vi "instrument_cluster.vi"() -> ()   [LabVIEW 2014]
uses:
  stateCtl.ctl
  <vilib>/Instr/_visa.llb/VISA Configure Serial Port (Instr).vi
  <vilib>/Utility/miscctls.llb/LVTextColorsTypeDef.ctl
  <vilib>/Utility/miscctls.llb/LVSelectionTypeDef.ctl
  <vilib>/Utility/miscctls.llb/LVFontTypeDef.ctl
  <vilib>/Utility/miscctls.llb/LVForegroundBackgroundColorsTypeDef.ctl
panel:
  out "S5":string
  out "S4":string
  out "S3":string
  out "S2":string
  out "S1":string
  out "S0":string
  in  "Text.Font 4":T1={"Font Name"="Arial", "Size"=0, "Bold"=FALSE, "Italic"=FALSE, "Underline"=FALSE, "Strikeout"=FALSE, "Color"=16776746}
  in  "Text.Text Colors 2":T2={"Text Color"=0, "Background Color"=3153414}
  in  "Text.Selection 2":T3
  in  "Text.Font 2":T1={"Font Name"="Arial", "Size"=55, "Bold"=FALSE, "Italic"=FALSE, "Underline"=FALSE, "Strikeout"=FALSE, "Color"=16776746}
  in  "Text.Colors 2":T4={"Foreground Color"=0, "Background Color"=3153414}
  in  "Text.Text Colors 3":T2={"Text Color"=0, "Background Color"=3153414}
  in  "Text.Selection 3":T3
  in  "Text.Font 3":T1={"Font Name"="Arial", "Size"=0, "Bold"=FALSE, "Italic"=FALSE, "Underline"=FALSE, "Strikeout"=FALSE, "Color"=16776746}
  in  "Text.Colors 3":T4={"Foreground Color"=0, "Background Color"=3153414}
  in  "Text.Colors":T4={"Foreground Color"=0, "Background Color"=3153414}
  in  "Text.Font":T1={"Font Name"="Arial", "Size"=15, "Bold"=FALSE, "Italic"=FALSE, "Underline"=FALSE, "Strikeout"=FALSE, "Color"=16776746}
  in  "Text.Selection":T3
  in  "Text.Text Colors":T2={"Text Color"=0, "Background Color"=3153414}
  out "exitLed":bool
  out "statusBar":string="     "
  in  "startButton":bool
  out "stopLed":bool
  out "startLed":bool
  in  "VISA Serial Port":refnum<visa-resource-name>
  in  "exitButton":bool
  in  "stopButton":bool
  # "String G"
  # "Gear String"
  # "Travelled Distance String"
  # "Pedal Position String"
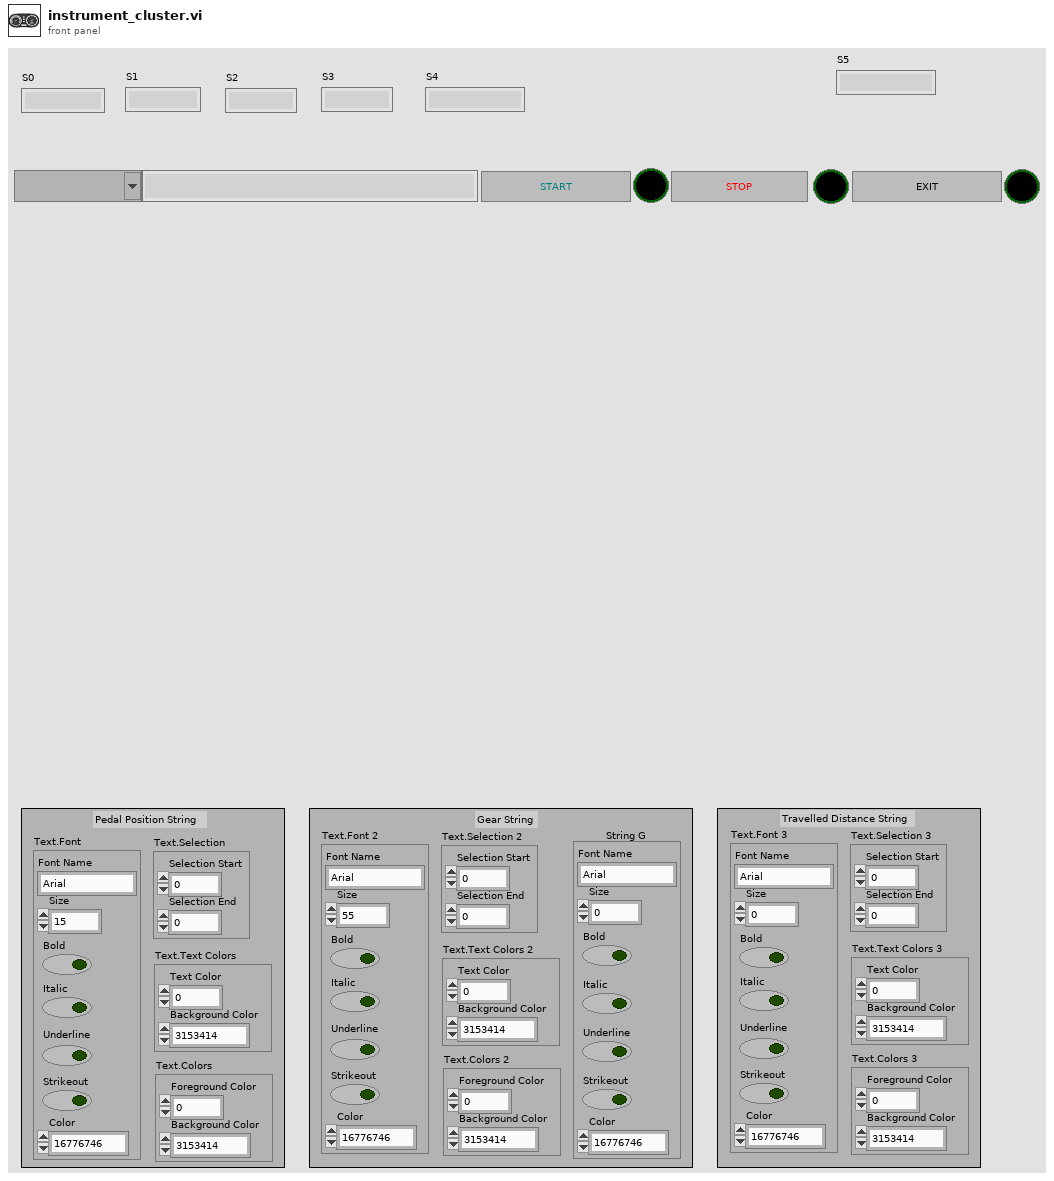
[diagram p1: front panel]
types:
  T1 = typedef "LVFontTypeDef.ctl" = cluster{"Font Name":string, "Size":u16, "Bold":bool, "Italic":bool, "Underline":bool, "Strikeout":bool, "Color":u32}
  T2 = typedef "LVTextColorsTypeDef.ctl" = cluster{"Text Color":u32, "Background Color":u32}
  T3 = typedef "LVSelectionTypeDef.ctl" = cluster{"Selection Start":u32, "Selection End":u32}
  T4 = typedef "LVForegroundBackgroundColorsTypeDef.ctl" = cluster{"Foreground Color":u32, "Background Color":u32}
  T5 = typedef "stateCtl.ctl" = enum16{"init", "ready", "running", "stopped", "exit"}
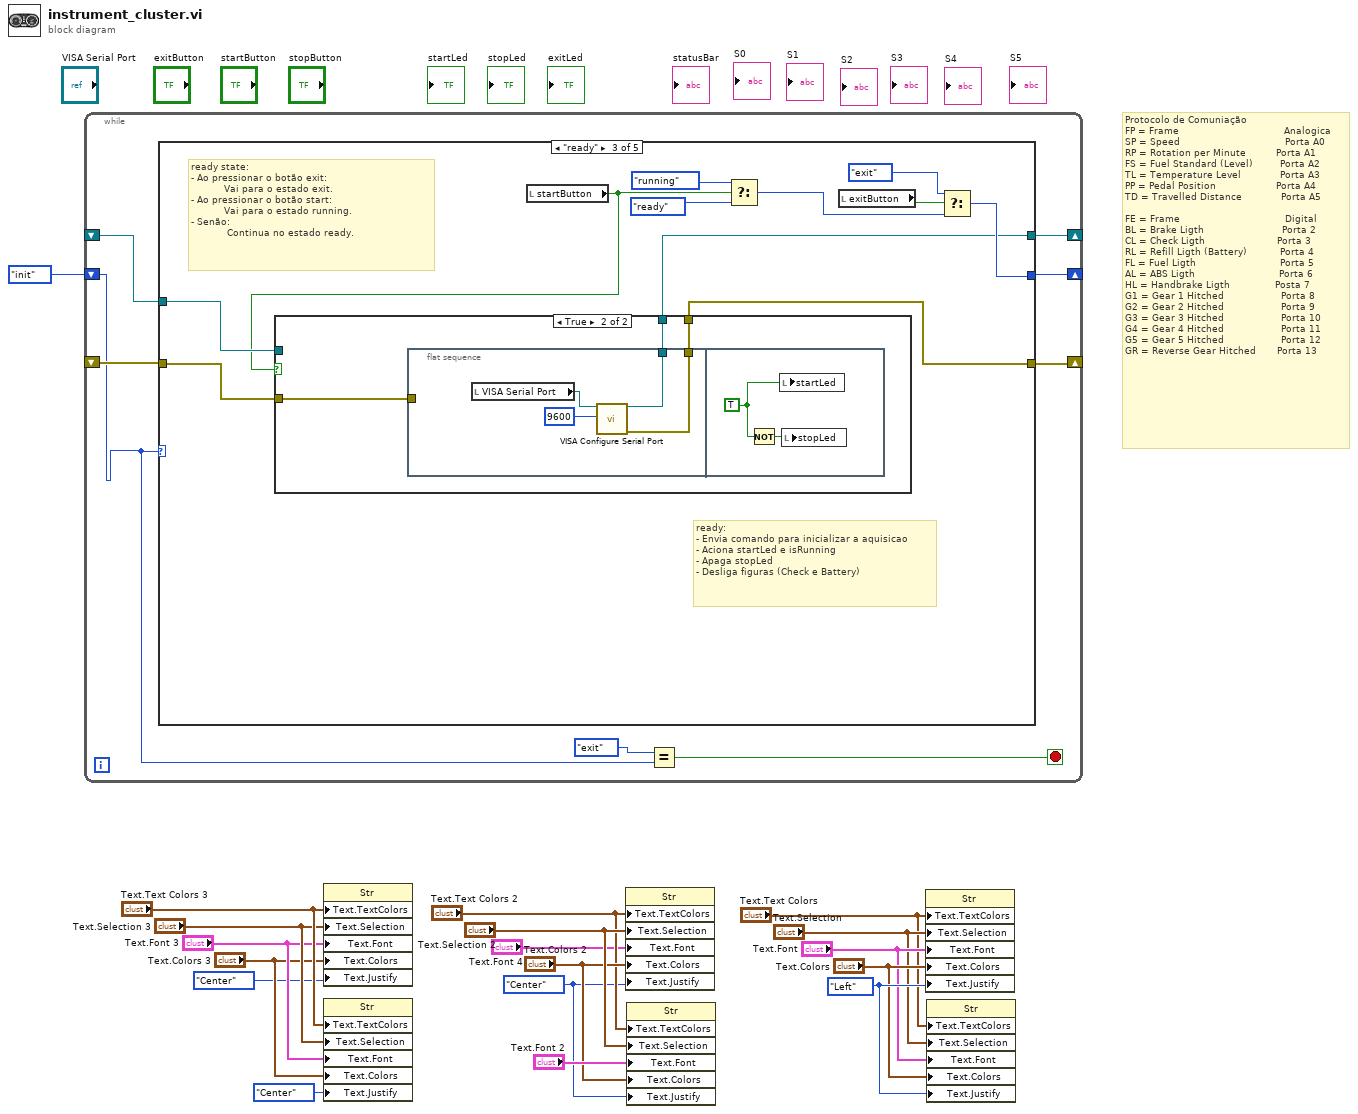
[diagram p0: block diagram]
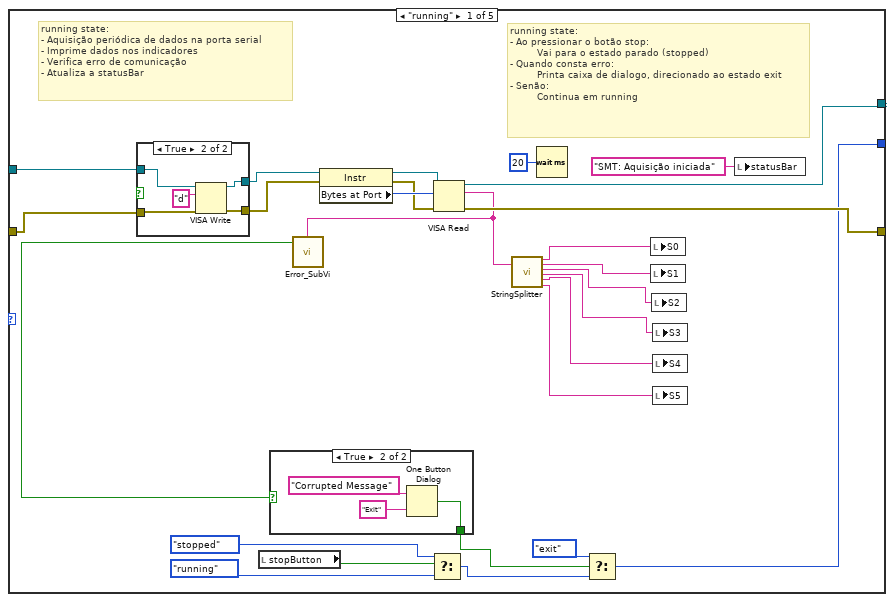
[diagram p2: hidden frame]
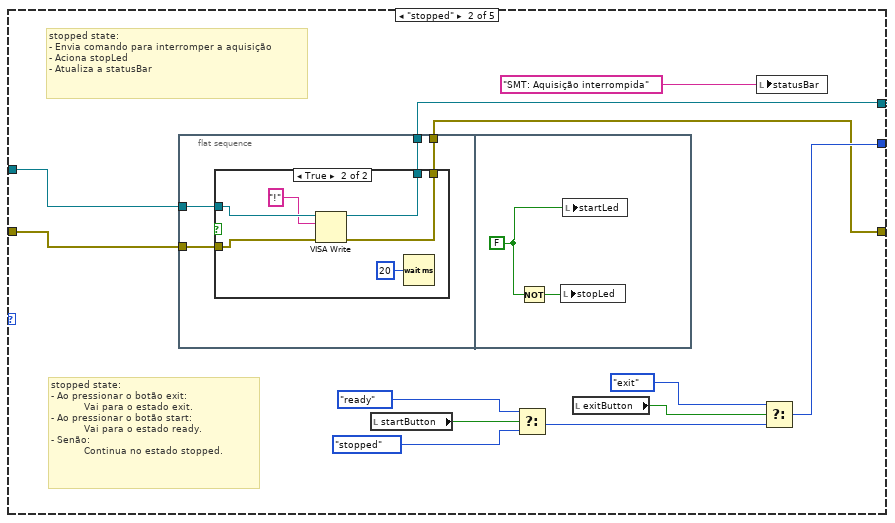
[diagram p5: hidden frame]
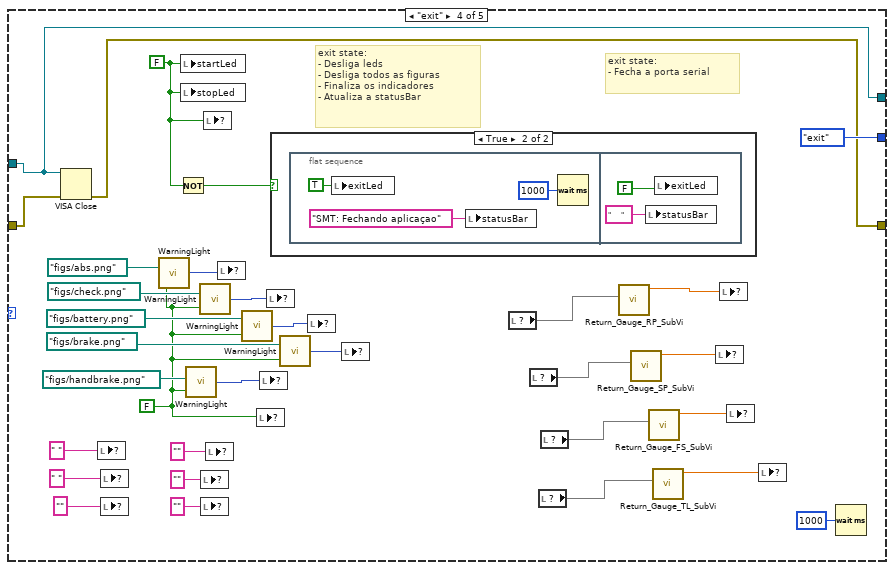
[diagram p8: hidden frame]
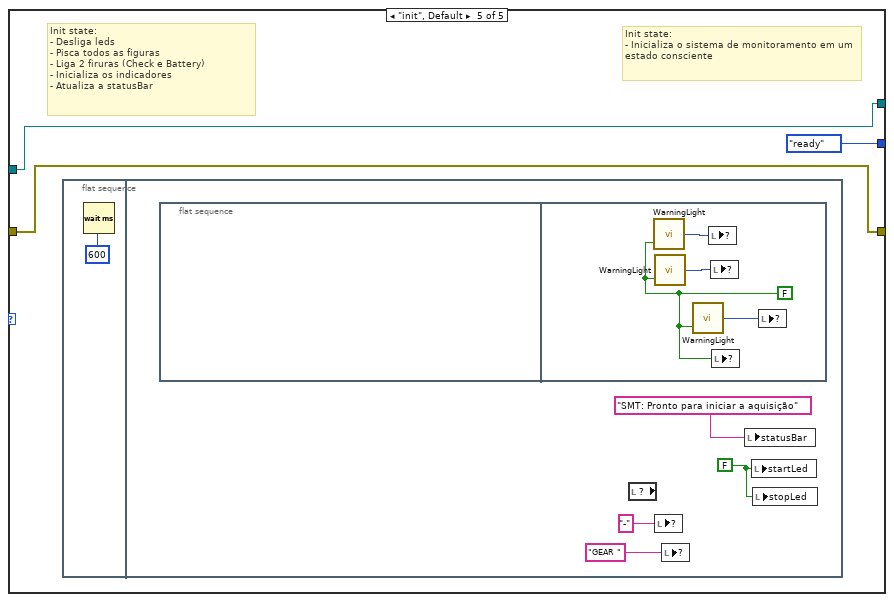
[diagram p10: hidden frame]
diagram:
  w1 = enum16{"Left", "Center", "Right"}."Center" ("Text.Justification")
  w23 = enum16{"Left", "Center", "Right"}."Left" ("Text.Justification")
  # "Protocolo de Comuniação \nFP = Frame                                   Analogica  \nSP = Speed                                   Porta A0\nRP = Rotation per Minute          Porta A1\nFS = Fuel Standard (Level)         Porta A2\nTL = Temperature Level             Porta A3\nPP = Pedal Position                    Porta A4\nTD = Travelled Distance             Porta A5\n\nFE = Frame                                   Digital \nBL = Brake Ligth                          Porta 2 \nCL = Check Ligth                        Porta 3\nRL = Refill Ligth (Battery)           Porta 4\nFL = Fuel Ligth                            Porta 5 \nAL = ABS Ligth                            Porta 6\nHL = Handbrake Ligth               Posta 7\nG1 = Gear 1 Hitched                   Porta 8\nG2 = Gear 2 Hitched                   Porta 9\nG3 = Gear 3 Hitched                   Porta 10\nG4 = Gear 4 Hitched                   Porta 11\nG5 = Gear 5 Hitched                   Porta 12\nGR = Reverse Gear Hitched       Porta 13"
  n1 = while {
    shift-right: [w27] -> _
    shift-left: _ -> [w31]
    shift-right: [w32] -> _
    shift-left: _ -> [w30]
    shift-right: [w28] -> _
    shift-left: stateCtl."init" ("state") -> [w25]
    stop <- w26 stop-if-true
    n2 = case shown="\"ready\"" w25 {
      tunnel: [w51 w74 w98 w150 w160] -> w27
      tunnel: [w50 w75 w97 w151 w159] -> w32
      tunnel: [w43 w79 w101 stateCtl."exit" ("state") stateCtl."ready" ("state")] -> w28
      tunnel: w31 -> [w45 w77 w99 w150 w160]
      tunnel: w30 -> [w46 w76 w100 w152 w159]
      frame "running" {
        # "running state:\n- Ao pressionar o botão stop: \n         Vai para o estado parado (stopped)\n- Quando consta erro:\n         Printa caixa de dialogo, direcionado ao estado exit  \n- Senão:          \n         Continua em running"
        # "running state:\n- Aquisição periódica de dados na porta serial\n- Imprime dados nos indicadores\n- Verifica erro de comunicação\n- Atualiza a statusBar"
        n3 = case shown="True" {
          selector: _ -> [_ _]
          tunnel: [w64 w68] -> w48
          tunnel: [w63 w67] -> w47
          tunnel: w46 -> [w64 w66]
          tunnel: w45 -> [w63 w65]
          frame False {
          }
          frame True {
            n4 = VISA Write(VISA resource name=w65, write buffer="d", error in (no error)=w66) -> (VISA resource name out=w67:refnum<visa-resource-name>, error out=w68:errorcluster)  [unwired: 1 out]
          }
        }
        n5 = local read "stopButton"() -> (w56:bool)
        n6 = property class="Instr"(reference=w47, error in=w48) -> (reference out=w52:refnum<visa-resource-name>, error out=w53:errorcluster, "Bytes at Port"=w54:u32)
        n7 = Select(t=stateCtl."stopped" ("state"), s=w56, f=stateCtl."running" ("state")) -> (s? t:f=w42:T5)
        n8 = VISA Read(VISA resource name=w52, byte count=w54, error in (no error)=w53) -> (VISA resource name out=w51:refnum<visa-resource-name>, read buffer=w39:string, error out=w50:errorcluster)  [unwired: 1 out]
        n9 = call "Error_SubVi.vi"("string"=w39) -> ("error"=w40:bool)  [unwired: 10 in]
        n10 = case shown="True" w40 {
          selector: w40 -> [w59 _]
          tunnel: [w59 w60] -> w41
          frame False {
          }
          frame True {
            n11 = One Button Dialog(message="Corrupted Message", button name ("OK")="Exit") -> (true=w60:bool)
          }
        }
        n12 = call "StringSplitter.vi"("Input String"=w39) -> ("S0"=w38:string, "S1"=w37:string, "S2"=w36:string, "S3"=w35:string, "S4"=w34:string, "S5"=w33:string)  [unwired: 13 in]
        n13 = Wait (ms)(milliseconds to wait=u32 20) -> ()  [unwired: 1 out]
        n14 = Select(t=stateCtl."exit" ("state"), s=w41, f=w42) -> (s? t:f=w43:T5)
        n15 = local write "S0"(w38) -> ()
        n16 = local write "S1"(w37) -> ()
        n17 = local write "S2"(w36) -> ()
        n18 = local write "S3"(w35) -> ()
        n19 = local write "S4"(w34) -> ()
        n20 = local write "S5"(w33) -> ()
        n21 = local write "statusBar"("SMT: Aquisição iniciada" ("statusBar")) -> ()
      }
      frame "stopped" {
        # "stopped state:\n- Ao pressionar o botão exit: \n           Vai para o estado exit.\n- Ao pressionar o botão start:\n           Vai para o estado ready.\n- Senão:\n           Continua no estado stopped."
        # "stopped state:\n- Envia comando para interromper a aquisição\n- Aciona stopLed\n- Atualiza a statusBar"
        n22 = flat-sequence {
          tunnel: w77 -> [w85]
          tunnel: w76 -> [w84]
          tunnel: [w83] -> w75
          tunnel: [w82] -> w74
          frame #0 {
            n23 = case shown="True" {
              selector: _ -> [_ _]
              tunnel: w85 -> [w87 w93]
              tunnel: w84 -> [w86 w92]
              tunnel: [w86 w88] -> w83
              tunnel: [w87 w90] -> w82
              frame False {
              }
              frame True {
                n24 = VISA Write(VISA resource name=w93, write buffer="!", error in (no error)=w92) -> (VISA resource name out=w90:refnum<visa-resource-name>, error out=w88:errorcluster)  [unwired: 1 out]
                n25 = Wait (ms)(milliseconds to wait=u32 20) -> ()  [unwired: 1 out]
              }
            }
          }
          frame #1 {
            w95 = FALSE ("Boolean")
            n26 = Not(x=w95) -> (.not. x?=w94:bool)
            n27 = local write "stopLed"(w94) -> ()
            n28 = local write "startLed"(w95) -> ()
          }
        }
        n29 = local read "startButton"() -> (w73:bool)
        n30 = Select(t=stateCtl."ready" ("state"), s=w73, f=stateCtl."stopped" ("state")) -> (s? t:f=w80:T5)
        n31 = local read "exitButton"() -> (w72:bool)
        n32 = local write "statusBar"("SMT: Aquisição interrompida" ("statusBar")) -> ()
        n33 = Select(t=stateCtl."exit" ("state"), s=w72, f=w80) -> (s? t:f=w79:T5)
      }
      frame "ready" {
        # "ready state:\n- Ao pressionar o botão exit: \n           Vai para o estado exit.\n- Ao pressionar o botão start:\n           Vai para o estado running.\n- Senão:\n            Continua no estado ready."
        # "ready:\n- Envia comando para inicializar a aquisicao\n- Aciona startLed e isRunning\n- Apaga stopLed\n- Desliga figuras (Check e Battery)"
        n34 = local read "startButton"() -> (w96:bool)
        n35 = case shown="True" w96 {
          tunnel: [w108 w109] -> w98
          tunnel: [w107 w110] -> w97
          tunnel: w99 -> [w108 _]
          tunnel: w100 -> [w107 w111]
          frame False {
          }
          frame True {
            n36 = flat-sequence {
              tunnel: w111 -> [_]
              tunnel: [w113] -> w110
              tunnel: [w112] -> w109
              frame #0 {
                n37 = local read "VISA Serial Port"() -> (w114:refnum<visa-resource-name>)
                n38 = call-poly "VISA Configure Serial Port"("VISA resource name"=w114, "baud rate (9600)"=u32 9600) -> ("VISA resource name out"=w112:refnum<visa-resource-name>, "error out"=w113:errorcluster)  [unwired: 12 in]
              }
              frame #1 {
                w117 = TRUE ("Boolean")
                n39 = Not(x=w117) -> (.not. x?=w116:bool)
                n40 = local write "startLed"(w117) -> ()
                n41 = local write "stopLed"(w116) -> ()
              }
            }
          }
        }
        n42 = Select(t=stateCtl."running" ("state"), s=w96, f=stateCtl."ready" ("state")) -> (s? t:f=w102:T5)
        n43 = local read "exitButton"() -> (w104:bool)
        n44 = Select(t=stateCtl."exit" ("state"), s=w104, f=w102) -> (s? t:f=w101:T5)
      }
      frame "exit" {
        w124 = FALSE
        w141 = FALSE ("startLed")
        # "exit state:\n- Desliga leds\n- Desliga todos as figuras\n- Finaliza os indicadores\n- Atualiza a statusBar"
        # "exit state:\n- Fecha a porta serial"
        n45 = VISA Close(VISA resource name=w150, error in (no error)=w152) -> (error out=w151:errorcluster)
        n46 = local write item#-1(" " ("String Gear")) -> ()
        n47 = local write item#-1(" " ("String TD")) -> ()
        n48 = local write item#-1("" ("String PP")) -> ()
        n49 = call "WarningLight.vi"("Boolean"=w124, "Path"=path "figs/abs.png" ("path to PNG file")) -> ("new picture"=w145:picture)
        n50 = Not(x=w141) -> (.not. x?=w142:bool)
        n51 = local write "startLed"(w141) -> ()
        n52 = local write "stopLed"(w141) -> ()
        n53 = call "WarningLight.vi"("Boolean"=w124, "Path"=path "figs/handbrake.png" ("path to PNG file")) -> ("new picture"=w132:picture)
        n54 = call "WarningLight.vi"("Boolean"=w124, "Path"=path "figs/check.png" ("path to PNG file")) -> ("new picture"=w146:picture)
        n55 = local write item#-1("" ("TD")) -> ()
        n56 = local write item#-1("" ("pedalPosition")) -> ()
        n57 = local write item#-1(w141) -> ()
        n58 = local write item#-1("" ("Gear")) -> ()
        n59 = local write item#-1(w145) -> ()
        n60 = call "WarningLight.vi"("Boolean"=w124, "Path"=path "figs/battery.png" ("path to PNG file")) -> ("new picture"=w147:picture)
        n61 = local write item#-1(w124) -> ()
        n62 = local write item#-1(w132) -> ()
        n63 = local write item#-1(w146) -> ()
        n64 = case shown="True" w142 {
          frame False {
          }
          frame True {
            n65 = flat-sequence {
              frame #0 {
                n66 = local write "exitLed"(TRUE ("exitLed")) -> ()
                n67 = local write "statusBar"("SMT: Fechando aplicaçao" ("statusBar")) -> ()
                n68 = Wait (ms)(milliseconds to wait=u32 1000) -> ()  [unwired: 1 out]
              }
              frame #1 {
                n69 = local write "statusBar"("     " ("statusBar")) -> ()
                n70 = local write "exitLed"(FALSE ("exitLed")) -> ()
              }
            }
          }
        }
        n71 = call "WarningLight.vi"("Boolean"=w124, "Path"=path "figs/brake.png" ("path to PNG file")) -> ("new picture"=w148:picture)
        n72 = local write item#-1(w147) -> ()
        n73 = local write item#-1(w148) -> ()
        n74 = local read item#-1() -> (w139)
        n75 = local read item#-1() -> (w136)
        n76 = local read item#-1() -> (w127)
        n77 = local read item#-1() -> (w130)
        n78 = call "Return_Gauge_RP_SubVi.vi"("number"=w139) -> ("Gauge"=w138:dbl, "Knob in"=w137:refnum<vi>)  [unwired: 9 in]
        n79 = call "Return_Gauge_SP_SubVi.vi"("number"=w136) -> ("Gauge"=w135:dbl, "Knob in"=w134:refnum<vi>)  [unwired: 9 in]
        n80 = call "Return_Gauge_FS_SubVi.vi"("number"=w130) -> ("Gauge"=w129:dbl, "Knob in"=w125:refnum<vi>)  [unwired: 9 in]
        n81 = call "Return_Gauge_TL_SubVi.vi"("number"=w127) -> ("Gauge"=w128:dbl, "Knob in"=w126:refnum<vi>)  [unwired: 9 in]
        n82 = local write item#-1(w135) -> ()
        n83 = local write item#-1(w138) -> ()
        n84 = local write item#-1(w129) -> ()
        n85 = local write item#-1(w128) -> ()
        n86 = Wait (ms)(milliseconds to wait=u32 1000) -> ()  [unwired: 1 out]
      }
      frame "init", Default {
        # "Init state:\n- Inicializa o sistema de monitoramento em um estado consciente"
        # "Init state:\n- Desliga leds\n- Pisca todos as figuras\n- Liga 2 firuras (Check e Battery)\n- Inicializa os indicadores\n- Atualiza a statusBar"
        n87 = flat-sequence {
          frame #0 {
            n88 = Wait (ms)(milliseconds to wait=u32 600) -> ()  [unwired: 1 out]
          }
          frame #1 {
            w167 = FALSE
            n89 = flat-sequence {
              frame #0 {
              }
              frame #1 {
                w168 = FALSE
                n90 = call "WarningLight.vi"("Boolean"=w168) -> ("new picture"=w173:picture, "Path"=w174:path)
                n91 = call "WarningLight.vi"("Boolean"=w168) -> ("new picture"=w172:picture, "Path"=w171:path)
                n92 = call "WarningLight.vi"("Boolean"=w168) -> ("new picture"=w169:picture, "Path"=w170:path)
                n93 = local write item#-1(w173) -> ()
                n94 = local write item#-1(w172) -> ()
                n95 = local write item#-1(w168) -> ()
                n96 = local write item#-1(w169) -> ()
              }
            }
            n97 = local read item#-1() -> (w165)
            n98 = local write item#-1("-" ("Gear")) -> ()
            n99 = local write item#-1("GEAR " ("String Gear")) -> ()
            n100 = local write "statusBar"("SMT: Pronto para iniciar a aquisição" ("statusBar")) -> ()
            n101 = local write "startLed"(w167) -> ()
            n102 = local write "stopLed"(w167) -> ()
          }
        }
      }
    }
    n103 = Equal?(x=stateCtl."exit" ("state"), y=w25) -> (x = y?=w26:bool)
  }
  n104 = property class="Str"("Text.TextColors"="Text.Text Colors 3", "Text.Selection"="Text.Selection 3", "Text.Font"="Text.Font 3", "Text.Colors"="Text.Colors 3", "Text.Justify"=enum16{"Left", "Center", "Right"}."Center" ("Text.Justification")) -> (reference=w9:refnum<vi>)  [unwired: 1 in, 2 out]
  n105 = property class="Str"("Text.TextColors"="Text.Text Colors 3", "Text.Selection"="Text.Selection 3", "Text.Font"="Text.Font 3", "Text.Colors"="Text.Colors 3", "Text.Justify"=enum16{"Left", "Center", "Right"}."Center" ("Text.Justification")) -> (reference=w4:refnum<vi>)  [unwired: 1 in, 2 out]
  n106 = property class="Str"("Text.TextColors"="Text.Text Colors 2", "Text.Selection"="Text.Selection 2", "Text.Font"="Text.Font 4", "Text.Colors"="Text.Colors 2", "Text.Justify"=w1) -> (reference=w8:refnum<vi>)  [unwired: 1 in, 2 out]
  n107 = property class="Str"("Text.TextColors"="Text.Text Colors 2", "Text.Selection"="Text.Selection 2", "Text.Font"="Text.Font 2", "Text.Colors"="Text.Colors 2", "Text.Justify"=w1) -> (reference=w7:refnum<vi>)  [unwired: 1 in, 2 out]
  n108 = property class="Str"("Text.TextColors"="Text.Text Colors", "Text.Selection"="Text.Selection", "Text.Font"="Text.Font", "Text.Colors"="Text.Colors", "Text.Justify"=w23) -> (reference=w6:refnum<vi>)  [unwired: 1 in, 2 out]
  n109 = property class="Str"("Text.TextColors"="Text.Text Colors", "Text.Selection"="Text.Selection", "Text.Font"="Text.Font", "Text.Colors"="Text.Colors", "Text.Justify"=w23) -> (reference=w5:refnum<vi>)  [unwired: 1 in, 2 out]
